vi "Read Output.vi"(8 "error in":errorcluster, 11 "4124 in":refnum<class "4124.lvclass">) -> (0 "error out":errorcluster, 2 "Output":bool, 3 "4124 out":refnum<class "4124.lvclass">)   [LabVIEW 2018, in "4124.lvlib" / "4124.lvclass"]
uses:
  4124.lvclass
  builds/Power_Supply.lvlibp/Power Supply.lvclass
  C:/Users/Ron.Dexter.LUMINARTECH/Desktop/builds/Power_Supply.lvlibp/Power Supply.lvclass
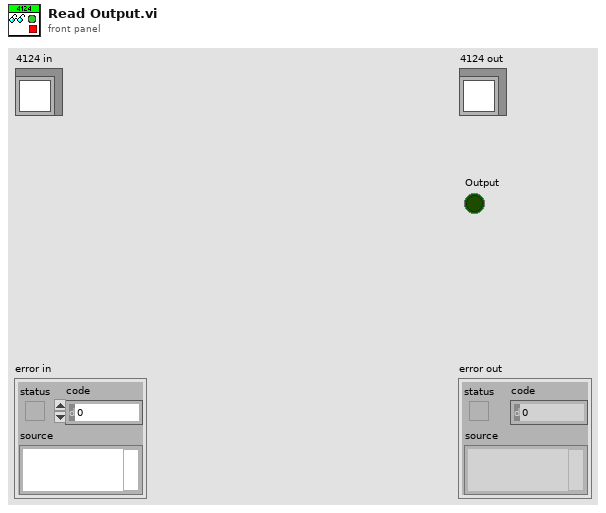
[diagram p1: front panel]
types:
  T1 = typedef "Power_Supply.lvlibp/Supply Settings.ctl" = cluster{"Voltage":dbl, "Current":dbl, "Output":bool}
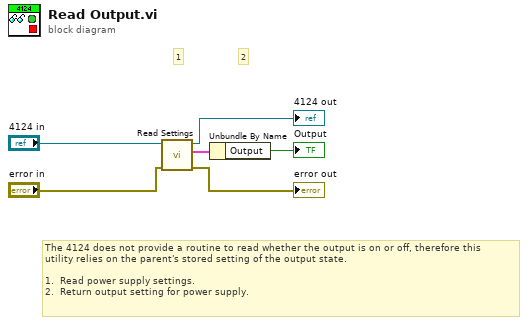
[diagram p0: block diagram]
diagram:
  # "The 4124 does not provide a routine to read whether the output is on or off, therefore this \nutility relies on the parent's stored setting of the output state.\n\n1.  Read power supply settings.\n2.  Return output setting for power supply."
  # "2"
  # "1"
  n1 = call "Read Settings.vi"("error in (no error)"="error in", "Power Supply in"="4124 in") -> ("error out"=→"error out":errorcluster, "Settings"=w2:T1, "Power Supply out"=→"4124 out":refnum<class "4124.lvclass">)  [unwired: 7 in]
  n2 = Unbundle By Name(w2) -> ("Output"=→"Output":bool)
